vi "Type of the message.vi"(8 "error in (no error)":errorcluster, 11 "RxTxCamera in":refnum<class "RxTxCamera.lvclass">) -> (0 "error out":errorcluster, 2 "Type":string, 3 "RxTxCamera out":refnum<class "RxTxCamera.lvclass">)   [LabVIEW 2018, in "RxTxCamera.lvclass"]
doc: "Este VI retorna a primeira linha da string da menssagem recebida, informando o tipo de dado que está chegando: comando, header, configuração ou status."
uses:
  RxTxCamera.lvclass
  C:/Users/Cliente/Desktop/Software Echarpe/RxTx/RxTx.lvclass
  RxTx/RxTx.lvclass/RxTx.ctl
  RxTx/RxTx.lvclass
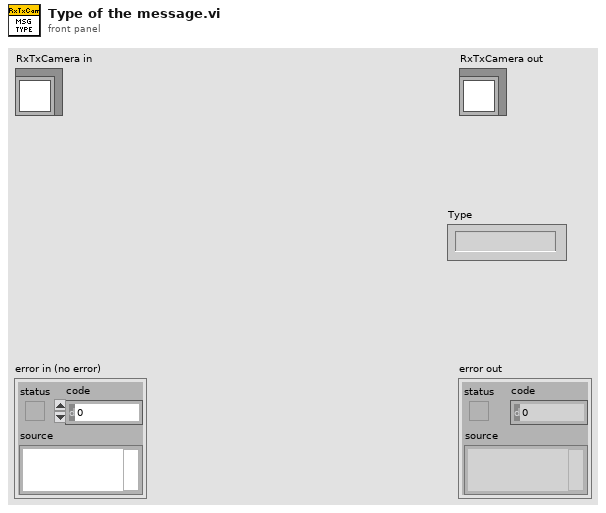
[diagram p1: front panel]
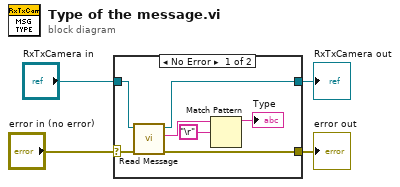
[diagram p0: block diagram]
diagram:
  n1 = case shown="No Error" "error in (no error)" {
    selector: "error in (no error)" -> [w7 w13]
    tunnel: [w6 w13] -> w3
    tunnel: [w8 w12] -> w1
    tunnel: "RxTxCamera in" -> [w9 w12]
    frame No Error {
      n2 = call "Read Message.vi"("error in (no error)"=w7, "RxTx in"=w9) -> ("error out"=w6:errorcluster, "Message"=w5:string, "RxTx out"=w8:refnum<class "RxTxCamera.lvclass">)  [unwired: 7 in]
      n3 = Match Pattern(string=w5, regular expression="\r") -> (before substring=→"Type":string)  [unwired: 1 in, 3 out]
    }
    frame Error {
    }
  }
  "error out" <- w3
  "RxTxCamera out" <- w1
